vi "Pulse Train Interp.vi"(6 "ntimes":i32=1, 7 "method":i32(ring)=1 items=["nearest", "linear", "spline", "cubic Hermite"], 8 "X is monotonic":bool, 9 "Xi":dbl[](array[numeric]) format="%_6g", 10 "X":dbl[](array[numeric]) format="%_6g", 11 "Y":dbl[](array[numeric]) format="%_6g") -> (0 "error":i32, 2 "xi used":dbl[](array[numeric]) format="%_6g", 3 "Yi":dbl[](array[numeric]))   [LabVIEW 2017, in "NI_AALBase.lvlib"]
uses:
  NI_AALBase.lvlib
  NI_Gmath.lvlib
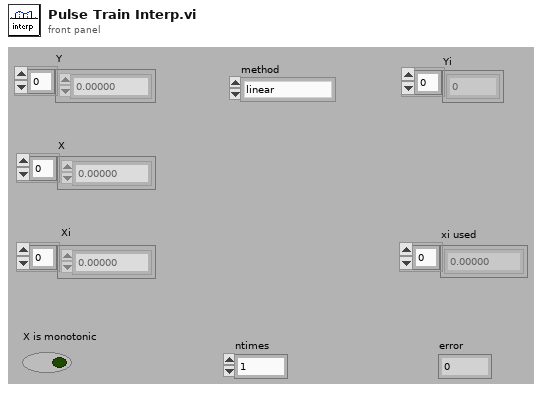
[diagram p1: front panel]
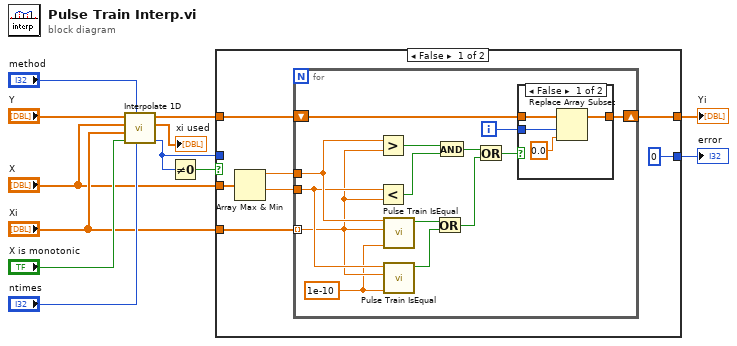
[diagram p0: block diagram]
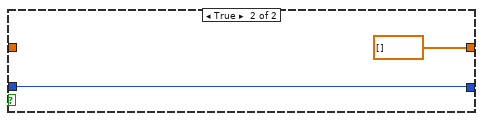
[diagram p3: hidden frame]
diagram:
  n1 = call "Interpolate 1D.vi"("ntimes"="ntimes", "method"="method", "X is monotonic"="X is monotonic", "xi"="Xi", "X"="X", "Y"="Y") -> ("error"=w1:i32, "xi used"=→"xi used":dbl[], "yi"=w8:dbl[])  [unwired: 3 in]
  n2 = Not Equal To 0?(x=w1) -> (x != 0?=w3:bool)
  n3 = case shown="False" w3 {
    tunnel: w8 -> [w19 _]
    tunnel: "Xi" -> [w18 _]
    tunnel: "X" -> [w17 _]
    tunnel: [w14 dbl[] []] -> w5
    tunnel: [0 w39] -> w2
    tunnel: w1 -> [_ w39]
    frame False {
      n4 = Array Max & Min(array=w17) -> (max value=w16:dbl, min value=w15:dbl)  [unwired: 2 out]
      n5 = for {
        tunnel: w18 -> [w26] mode=indexing
        tunnel: w16 -> [w28]
        tunnel: w15 -> [w27]
        shift-right: [w33] -> w14
        shift-left: w19 -> [w30]
        i -> [w29]
        w20 = 1e-10 ("y")
        n6 = Greater?(x=w28, y=w26) -> (0:w32:bool)
        n7 = Less?(x=w27, y=w26) -> (x < y?=w31:bool)
        n8 = call "Pulse Train IsEqual.vi"("related precise"=w20, "x2"=w26, "x1"=w28) -> ("x1 = x2?"=w25:bool)  [unwired: 8 in]
        n9 = call "Pulse Train IsEqual.vi"("related precise"=w20, "x2"=w26, "x1"=w27) -> ("x1 = x2?"=w24:bool)  [unwired: 8 in]
        n10 = Or(x=w25, y=w24) -> (x .or. y?=w22:bool)
        n11 = And(x=w32, y=w31) -> (x .and. y?=w23:bool)
        n12 = Or(x=w23, y=w22) -> (x .or. y?=w21:bool)
        n13 = case shown="False" w21 {
          tunnel: w30 -> [w37 w38]
          tunnel: w29 -> [w35 _]
          tunnel: [w36 w38] -> w33
          frame False {
            n14 = Replace Array Subset(array=w37, new element=0.0 ("new element/subarray"), index=w35) -> (w36:dbl[])
          }
          frame True {
          }
        }
      }
    }
    frame True {
    }
  }
  "Yi" <- w5
  "error" <- w2
